vi "Command_Joint_Angles.vi"(0 "Side":T3, 1 "node":string, 2 "Arm Angles (degrees)":T2, 3 "error in":errorcluster, 4 "Mode":T1=1 items=["Position"=1, "Velocity"=2, "Effort"=3]) -> (6 "error out":errorcluster)   [LabVIEW 2010]
uses:
  <userlib>/ROSforLV/ROS/Code/SubVIs/BaxterSide.ctl
  <userlib>/ROSforLV/ROS/Code/SubVIs/BaxterArmsSmall.ctl
  <userlib>/ROSforLV/ROS/Code/SubVIs/JointMode.ctl
  <userlib>/ROSforLV/ROS/Code/Console/Servers/ServerSubs/TopicDef.ctl
  <userlib>/ROSforLV/ROS/Code/SubVIs/_ROSDirection.ctl
panel:
  out "Move Command":string
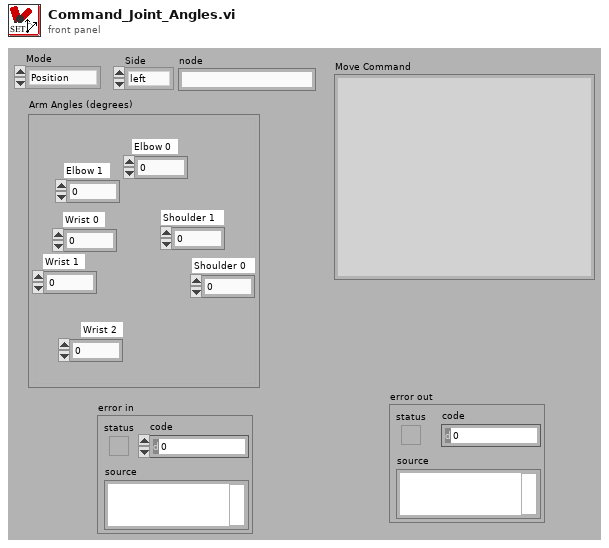
[diagram p1: front panel]
types:
  T1 = typedef "JointMode.ctl" = u8
  T2 = typedef "BaxterArmsSmall.ctl" = cluster{"Elbow 0":dbl, "Elbow 1":dbl, "Shoulder 0":dbl, "Shoulder 1":dbl, "Wrist 0":dbl, "Wrist 1":dbl, "Wrist 2":dbl}
  T3 = typedef "BaxterSide.ctl" = enum16{"left", "right"}
  T4 = typedef "TopicDef.ctl" = cluster{"Topic":string, "Type":string, "Action":T5, "Update (ms)":u16, "write queue":u16}
  T5 = typedef "_ROSDirection.ctl" = enum16{"Node", "Publisher", "Subscriber", "Service Client"}
  T6 = typedef "_ROSControl.ctl" = cluster{"topic port":u16, "Node":string, "topic":string, "type":string, "node port":u32, "error ":errorcluster, "Direction":T5, "APIs":string[], "Update (ms)":u16, "write queue":u16}
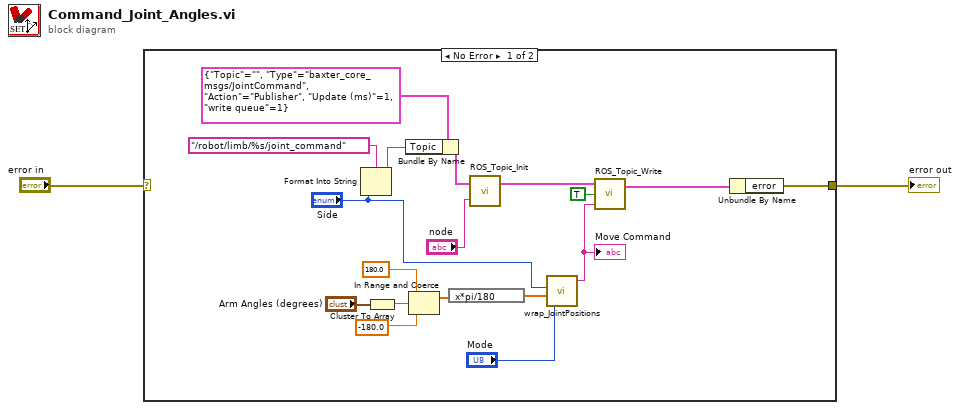
[diagram p0: block diagram]
diagram:
  n1 = case shown="No Error" "error in" {
    selector: "error in" -> [_ w21]
    tunnel: [w20 w21] -> w2
    frame No Error {
      n2 = Format Into String(format string="/robot/limb/%s/joint_command" ("Topic"), "Side") -> (resulting string=w6:string)  [unwired: 2 in, 1 out]
      n3 = Cluster To Array(cluster="Arm Angles (degrees)") -> (array=w15:dbl[])
      n4 = Bundle By Name(cluster=T4 {"Topic"="", "Type"="baxter_core_msgs/JointCommand", "Action"=enum."Publisher", "Update (ms)"=1, "write queue"=1} ("Definitions"), "Topic"=w6) -> (w3:T4)
      n5 = In Range and Coerce(upper limit=180.0 ("Elbow 0"), x=w15, lower limit=-180.0 ("Elbow 0")) -> (coerced(x)=w11:dbl[])  [unwired: 1 out]
      n6 = expression code="x*pi/180"(w11) -> (w10:dbl[])
      n7 = call <userlib>:"ROS_Topic_Init.vi"("node"="node", "Definitions"=w3) -> ("ROS out"=w18:T6)  [unwired: 1 in]
      n8 = call <userlib>:"wrap_JointPositions.vi"("Mode"="Mode", "Positions"=w10, "Side"="Side") -> ("msg out"=w12:string)  [unwired: 3 in]
      "Move Command" <- w12
      n9 = call <userlib>:"ROS_Topic_Write.vi"("Msg in"=w12, "Continuous?"=TRUE, "ROS in"=w18) -> ("ROS out"=w17:T6)  [unwired: 1 in]
      n10 = Unbundle By Name(w17) -> ("error"=w20:errorcluster)
    }
    frame Error {
    }
  }
  "error out" <- w2
